vi "linkToUI.vi"(8 "error in (no error)":errorcluster, 9 "Pane VI":string="AjustePrevio1.vi", 10 "subPanel":refnum<vi>, 11 "Usuario in":refnum<class "Aplicacion.lvclass">) -> (0 "error out":errorcluster, 3 "Ususario out":refnum<class "Aplicacion.lvclass">)   [LabVIEW 2019]
uses:
  User Interface/UI.lvclass
  PanelFactory/PanelFactory.lvclass
  Usuarios/Usuarios.lvclass
  Aplicacion.lvclass
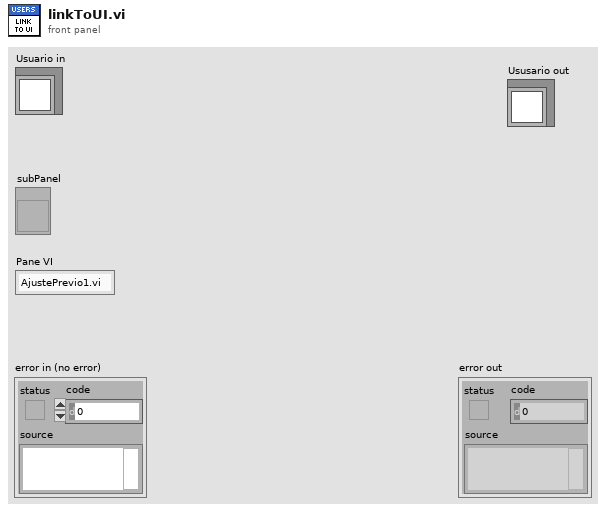
[diagram p1: front panel]
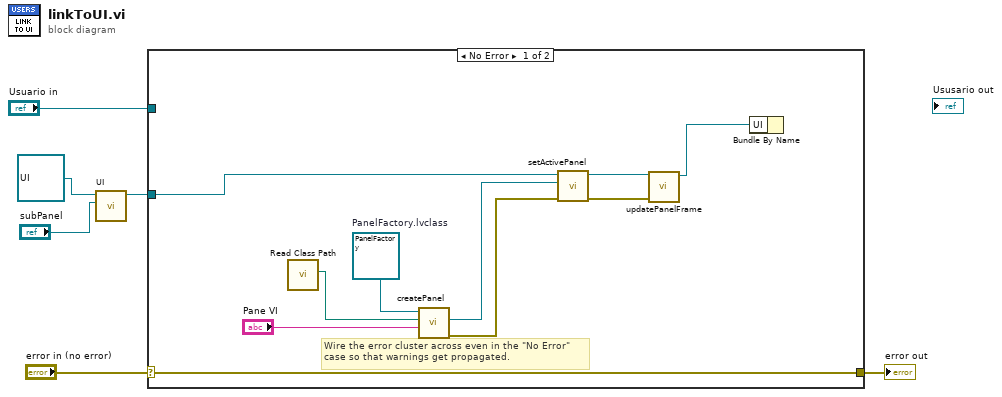
[diagram p0: block diagram]
diagram:
  n1 = call "UI.vi"("subPanel"="subPanel", "UI in"=refnum<class "UI.lvclass"> refnum ("UI.lvclass")) -> ("UI out"=w3:refnum<class "UI.lvclass">)  [unwired: 8 in, 1 out]
  n2 = case shown="No Error" "error in (no error)" {
    selector: "error in (no error)" -> [w17 w18]
    tunnel: [w17 w18] -> w5
    tunnel: "Usuario in" -> [w7 _]
    tunnel: w3 -> [w13 _]
    frame No Error {
      w16 = refnum<class "PanelFactory.lvclass"> refnum  # PanelFactory.lvclass
      # "Wire the error cluster across even in the \"No Error\"\ncase so that warnings get propagated."
      n3 = call-dynamic "Read Class Path.vi"() -> ("Class Path"=w8:path)  [unwired: 9 in, 2 out]
      n4 = call "createPanel.vi"("Pane VI"="Pane VI", "Path"=w8, "PanelFactory in"=w16) -> ("error out"=w14:errorcluster, "Panel out"=w15:refnum<class "Panel.lvclass">)  [unwired: 7 in]
      n5 = call "setActivePanel.vi"("error in (no error)"=w14, "Panel"=w15, "UI in"=w13) -> ("error out"=w11:errorcluster, "UI out"=w12:refnum<class "UI.lvclass">)  [unwired: 7 in]
      n6 = call "updatePanelFrame.vi"("error in (no error)"=w11, "UI in"=w12) -> ("UI out"=w10:refnum<class "UI.lvclass">)  [unwired: 8 in, 1 out]
      n7 = Bundle By Name("UI"=w10) -> ()  [unwired: 1 in, 1 out]
    }
    frame Error {
    }
  }
  "error out" <- w5
